vi "Main.vi"() -> ()   [LabVIEW 2026]
uses:
  <vilib>/ErrorRing/Error Ring.xnode
panel:
  in  "Main Tab Control":T1(tab)
  in  "Scan Information":T2 {"Date" format="%<%x>T"}
  in  "Calculated Diameter & Overscan Steps %":T3
  in  "Calculate Scan":bool
  in  "Scan Settings":T4
  in  "Transducer Information":string[][](table)
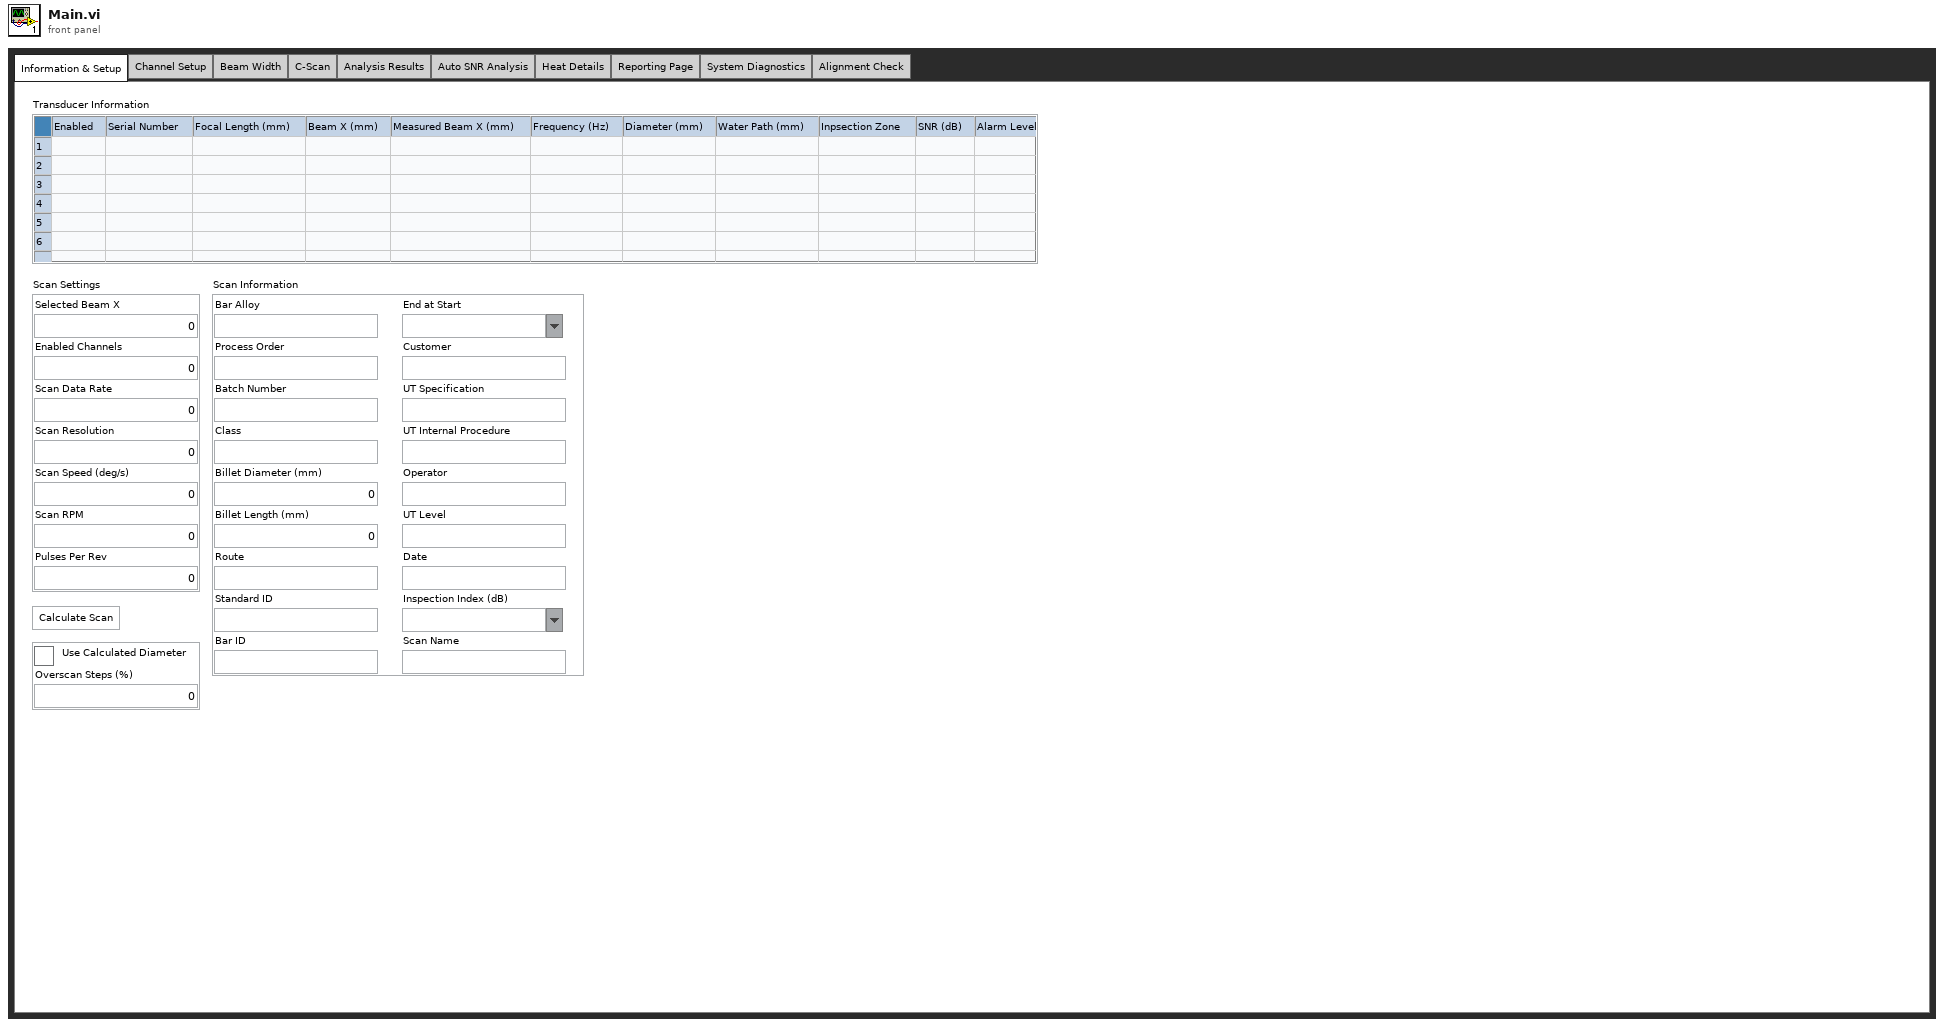
[diagram p1: front panel]
types:
  T1 = enum32{"Information & Setup", "Channel Setup", "Beam Width", "C-Scan", "Analysis Results", "Auto SNR Analysis", "Heat Details", "Reporting Page", "System Diagnostics", "Alignment Check"}
  T2 = cluster{"Bar ID":string, "Standard ID":string, "Route":string, "Billet Length (mm)":dbl, "Billet Diameter (mm)":dbl, "Class":string, "Batch Number":string, "Process Order":string, "Bar Alloy":string, "Scan Name":string, "Inspection Index (dB)":string, "Date":timestamp, "UT Level":string, "Operator":string, "UT Internal Procedure":string, "UT Specification":string, "Customer":string, "End at Start":string}
  T3 = cluster{"Use Calculated Diameter":bool, "Overscan Steps (%)":dbl}
  T4 = cluster{"Selected Beam X":dbl, "Enabled Channels":dbl, "Scan Data Rate":dbl, "Scan Resolution":dbl, "Scan Speed (deg/s)":dbl, "Scan RPM":dbl, "Pulses Per Rev":dbl}
  T5 = enum16{"Init", "Init Hardware", "Main", "Reset", "Error", "Shutdown"}
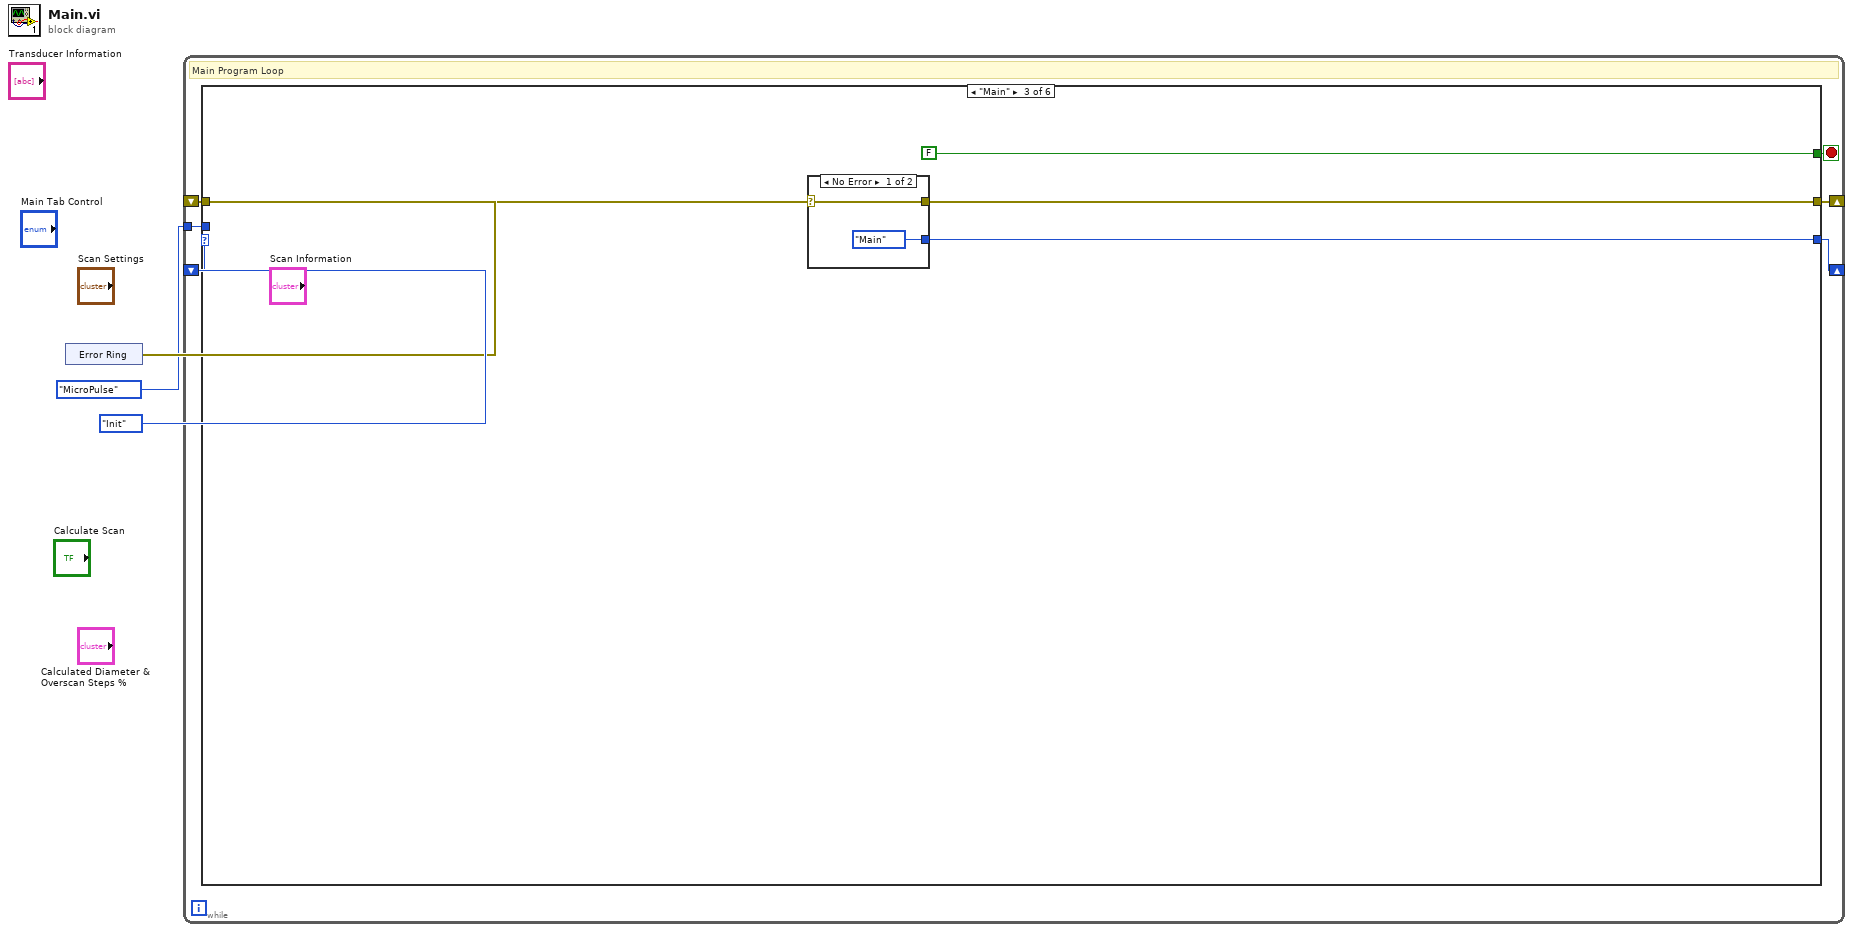
[diagram p0: block diagram]
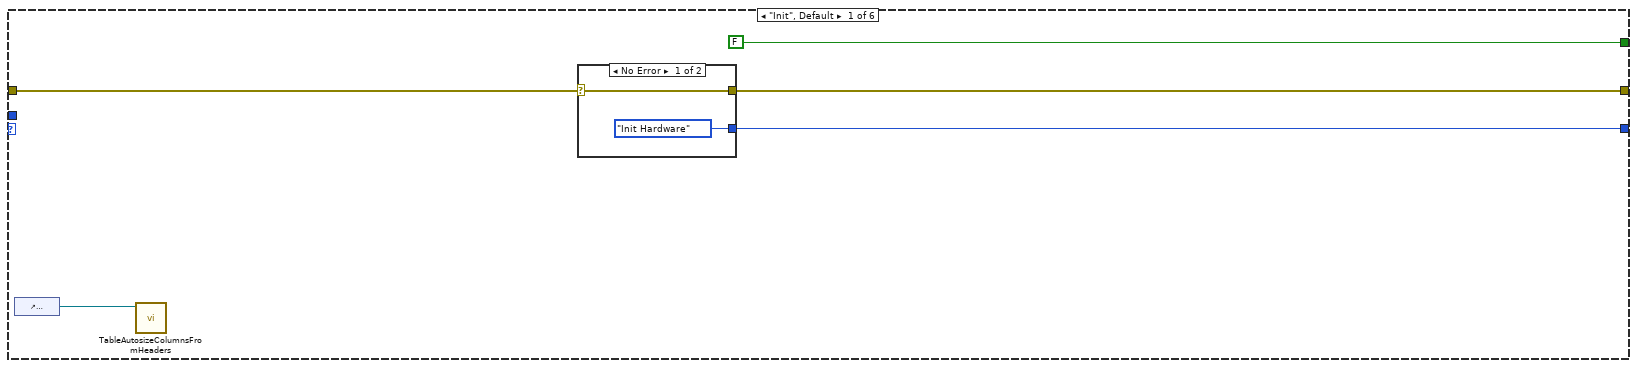
[diagram p2: hidden frame]
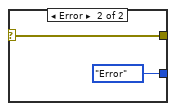
[diagram p3: hidden frame]
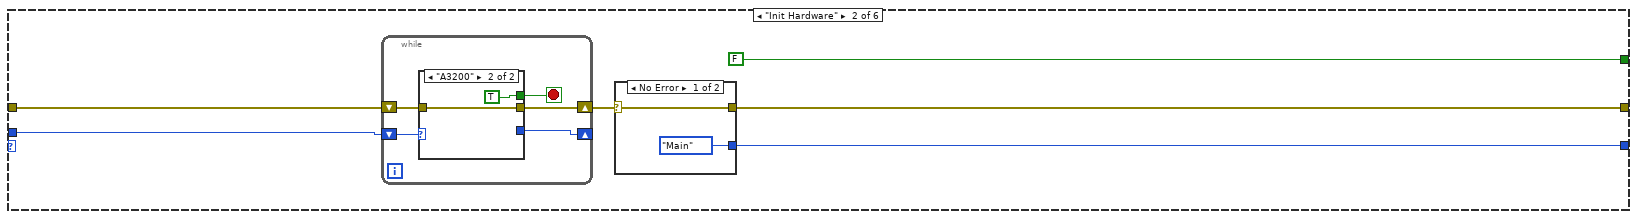
[diagram p4: hidden frame]
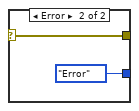
[diagram p5: hidden frame]
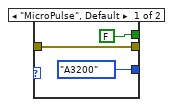
[diagram p6: hidden frame]
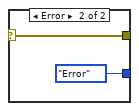
[diagram p7: hidden frame]
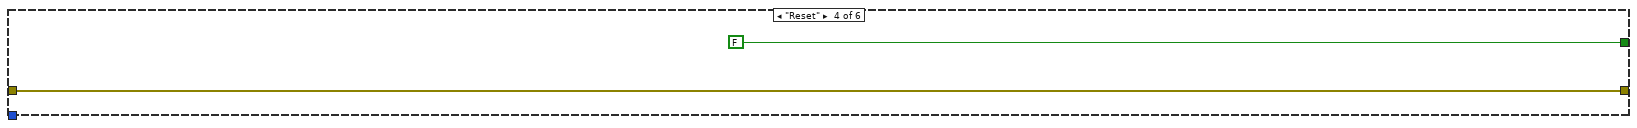
[diagram p8: hidden frame]
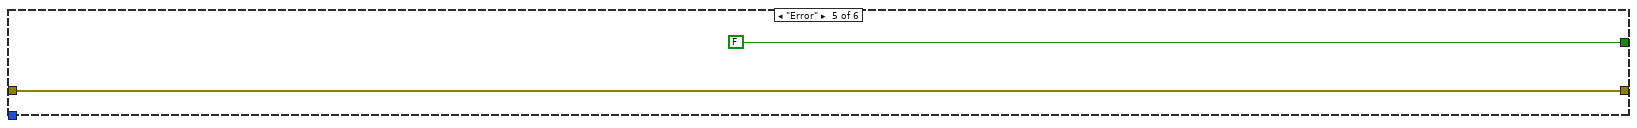
[diagram p9: hidden frame]
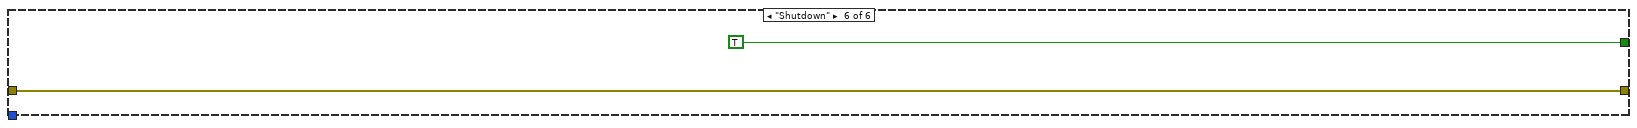
[diagram p10: hidden frame]
diagram:
  n1 = xnode "Error Ring"() -> ("error out"=w2:errorcluster)
  n2 = while {
    shift-right: [w6] -> _
    shift-left: T5."Init" -> [w9]
    shift-right: [w5] -> _
    shift-left: w2 -> [w8]
    tunnel: enum16{"MicroPulse", "A3200"}."MicroPulse" -> [w7]
    stop <- w4 stop-if-true
    # "Main Program Loop"
    n3 = case shown="\"Main\"" w9 {
      tunnel: w8 -> [w14 w23 w42 w48 w50 w52]
      tunnel: [w12 w21 w41 w48 w50 w52] -> w5
      tunnel: w7 -> [_ w24 _ _ _ _]
      tunnel: [w13 w20 w40 _ _ _] -> w6
      tunnel: [FALSE FALSE FALSE FALSE FALSE TRUE] -> w4
      frame "Init", Default {
        n4 = control-ref of="Transducer Information"() -> (w10:refnum<vi>)
        n5 = call "TableAutosizeColumnsFromHeaders.vi"("Table in"=w10) -> ()  [unwired: 11 in]
        n6 = case shown="No Error" w14 {
          selector: w14 -> [w16 w18]
          tunnel: [w16 w18] -> w12
          tunnel: [T5."Init Hardware" T5."Error"] -> w13
          frame No Error {
          }
          frame Error {
          }
        }
      }
      frame "Init Hardware" {
        n7 = while {
          shift-right: [w31] -> w22
          shift-left: w23 -> [w32]
          shift-right: [w29] -> _
          shift-left: w24 -> [w33]
          stop <- w30 stop-if-true
          n8 = case shown="\"A3200\"" w33 {
            tunnel: [w35 w38] -> w31
            tunnel: w32 -> [w35 w38]
            tunnel: [FALSE TRUE] -> w30
            tunnel: [enum16{"MicroPulse", "A3200"}."A3200" _] -> w29
            frame "MicroPulse", Default {
            }
            frame "A3200" {
            }
          }
        }
        n9 = case shown="No Error" w22 {
          selector: w22 -> [w26 w28]
          tunnel: [w26 w28] -> w21
          tunnel: [T5."Main" T5."Error"] -> w20
          frame No Error {
          }
          frame Error {
          }
        }
      }
      frame "Main" {
        n10 = case shown="No Error" w42 {
          selector: w42 -> [w44 w46]
          tunnel: [w44 w46] -> w41
          tunnel: [T5."Main" T5."Error"] -> w40
          frame No Error {
          }
          frame Error {
          }
        }
      }
      frame "Reset" {
      }
      frame "Error" {
      }
      frame "Shutdown" {
      }
    }
  }
